vi "XY Graph Get Deleted Cursor Index.vi"(8 "Error In":errorcluster, 9 "Old Cursor List":T1, 11 "XYGraph in":refnum<vi>) -> (0 "Error Out":errorcluster, 1 "New Cursor List":T1, 2 "Vertices":cluster{"X":dbl, "Y":dbl}[](array[cluster]), 3 "Deleted Cursor Index":i32)   [LabVIEW 2021, in "XY Graph Add-Ons.lvlib"]
doc: "This assumes that only one cursor was deleted"
uses:
  XY Graph Add-Ons.lvlib
  <vilib>/Utility/miscctls.llb/LVCursorListTypeDef.ctl
  <userlib>/_OpenG.lib/array/array.llb/Filter 1D Array (Variant)__ogtk.vi
  <userlib>/_OpenG.lib/array/array.llb/Filter 1D Array (I32)__ogtk.vi
  <userlib>/_OpenG.lib/array/array.llb/openg_array.lvlib
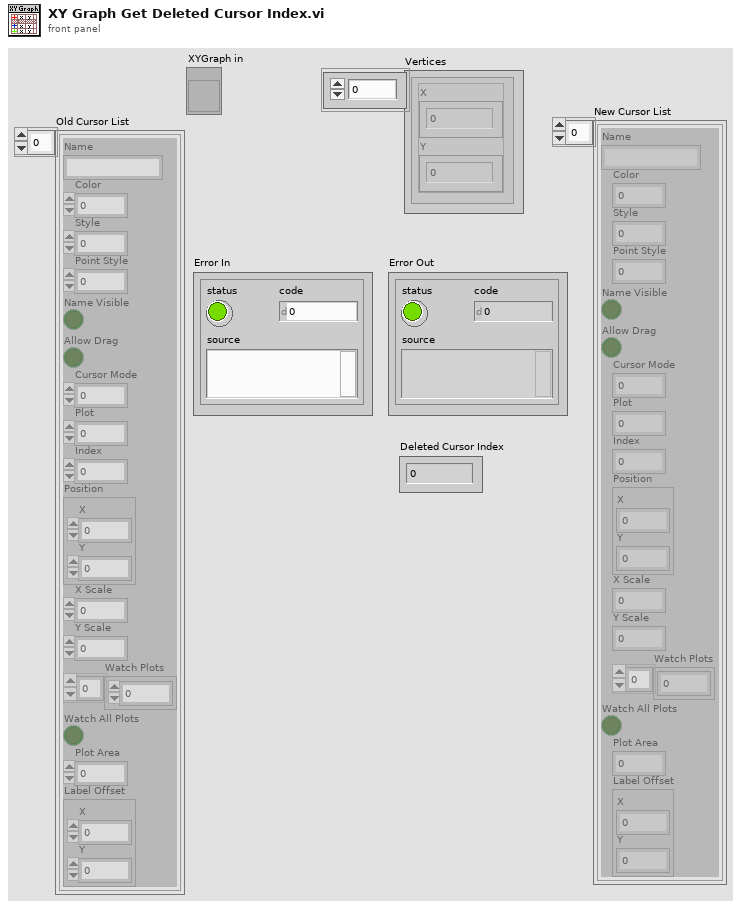
[diagram p1: front panel]
types:
  T1 = typedef "LVCursorListTypeDef.ctl" = cluster{"Name":string, "Color":u32, "Style":u8, "Point Style":u8, "Name Visible":bool, "Allow Drag":bool, "Cursor Mode":u32, "Plot":i32, "Index":i32, "Position":cluster{"X":dbl, "Y":dbl}, "X Scale":u32, "Y Scale":u32, "Watch Plots":i32[], "Watch All Plots":bool, "Plot Area":i32, "Label Offset":cluster{"X":dbl, "Y":dbl}}[]
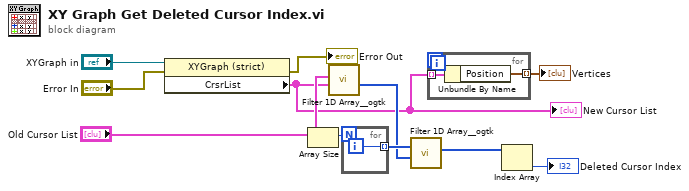
[diagram p0: block diagram]
diagram:
  n1 = property class="XYGraph (strict)"(reference="XYGraph in", error in="Error In") -> (error out=→"Error Out":errorcluster, "CrsrList"=w2:T1)  [unwired: 1 out]
  "New Cursor List" <- w2
  n2 = Array Size(array="Old Cursor List") -> (size(s)=w9:i32)
  n3 = call-poly <userlib>:"Filter 1D Array__ogtk.vi"("items to filter"=w2, "array"="Old Cursor List") -> ("filtered item indices"=w7:i32[])  [unwired: 4 in, 1 out]
  n4 = for {
    N: w9 -> [_]
    tunnel: [w12] -> w8 mode=indexing
    i -> [w12]
  }
  n5 = call-poly <userlib>:"Filter 1D Array__ogtk.vi"("items to filter"=w7, "array"=w8) -> ("filtered array"=w6:i32[])  [unwired: 4 in, 1 out]
  n6 = for {
    tunnel: w2 -> [w14] mode=indexing
    tunnel: [w13] -> w1 mode=indexing
    n7 = Unbundle By Name(w14) -> ("Position"=w13:cluster{"X":dbl, "Y":dbl})
  }
  "Vertices" <- w1
  n8 = Index Array(array=w6) -> (element=→"Deleted Cursor Index":i32)  [unwired: 1 in]
